vi "Method.vi"(4 "Value":refnum<class "Abs_Single Float.lvclass">) -> (1 "Result":refnum<class "Abs_Single Float.lvclass">)   [LabVIEW 2021, in "Increment_SGL.lvclass"]
uses:
  Increment_SGL.lvclass
  Abs_Types/Single Float/Abs_Single Float.lvclass
  C:/TSA/LV_Abstract/Source/Functions/Support/Function/One Terminal/SGL/AbsFunc_One Term_SGL.lvclass
  C:/Program Files (x86)/National Instruments/LabVIEW 2021/vi.lib/TSA/Abstract Data Classes/Abs_Types/Single Float/Abs_Single Float.lvclass
  Support/Function/One Terminal/SGL/AbsFunc_One Term_SGL.lvclass/AbsFunc_One Term_SGL.ctl
  Support/Function/One Terminal/SGL/Properties/Write Numeric A.vi
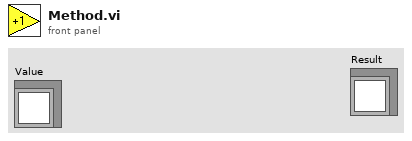
[diagram p1: front panel]
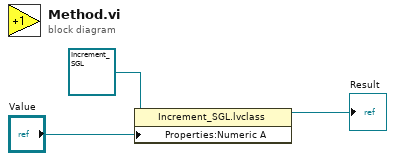
[diagram p0: block diagram]
diagram:
  n1 = property class="Increment_SGL.lvclass"(reference=refnum<class "Increment_SGL.lvclass"> refnum ("Decrement_DBL.lvclass"), "Properties:Numeric A"="Value") -> (reference out=→"Result":refnum<class "Increment_SGL.lvclass">)  [unwired: 1 in, 1 out]
